vi "LinearPlntInvFF_Calculate_NextR.vi"(9 "NextR":T1, 11 "Input Linear Plant Inv FF":T2) -> (0 "Error":bool, 2 "Uff":T1, 3 "Output Linear Plant Inv FF":T2)   [LabVIEW 2019, in "Trajectory_Library.lvlib"]
doc: "Creates a new LINEAR PLANT INVERSION FEEDFORWARD data cluster with the specified values. \n\n\nInputs: \n - XXX -- XXX.\n\nOutputs:\n - XXX -- XXX."
uses:
  LINEAR_PLANT_INV_FF.ctl
  <vilib>/Analysis/Matrix/Datatypes/RealMatrix.ctl
  Trajectory_Library.lvlib
  <vilib>/Analysis/Matrix/NI_Matrix.lvlib
panel:
  # "<States,1>"
  # "<Inputs,1>"
  # "<States,Inputs>"
  # "<States,States>"
  # "<States,1>"
  # "<Inputs,1>"
  # "<States,Inputs>"
  # "<States,States>"
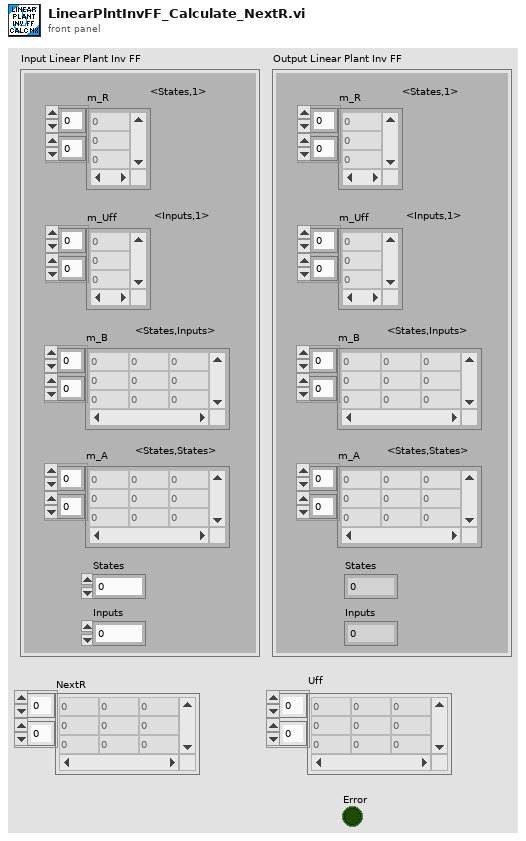
[diagram p1: front panel]
types:
  T1 = typedef "NI_Matrix.lvlib/RealMatrix.ctl" = dbl[][]
  T2 = typedef "Trajectory_Library.lvlib/LINEAR_PLANT_INV_FF.ctl" = cluster{"m_R":T1, "m_Uff":T1, "m_B":T1, "m_A":T1, "States":i32, "Inputs":i32}
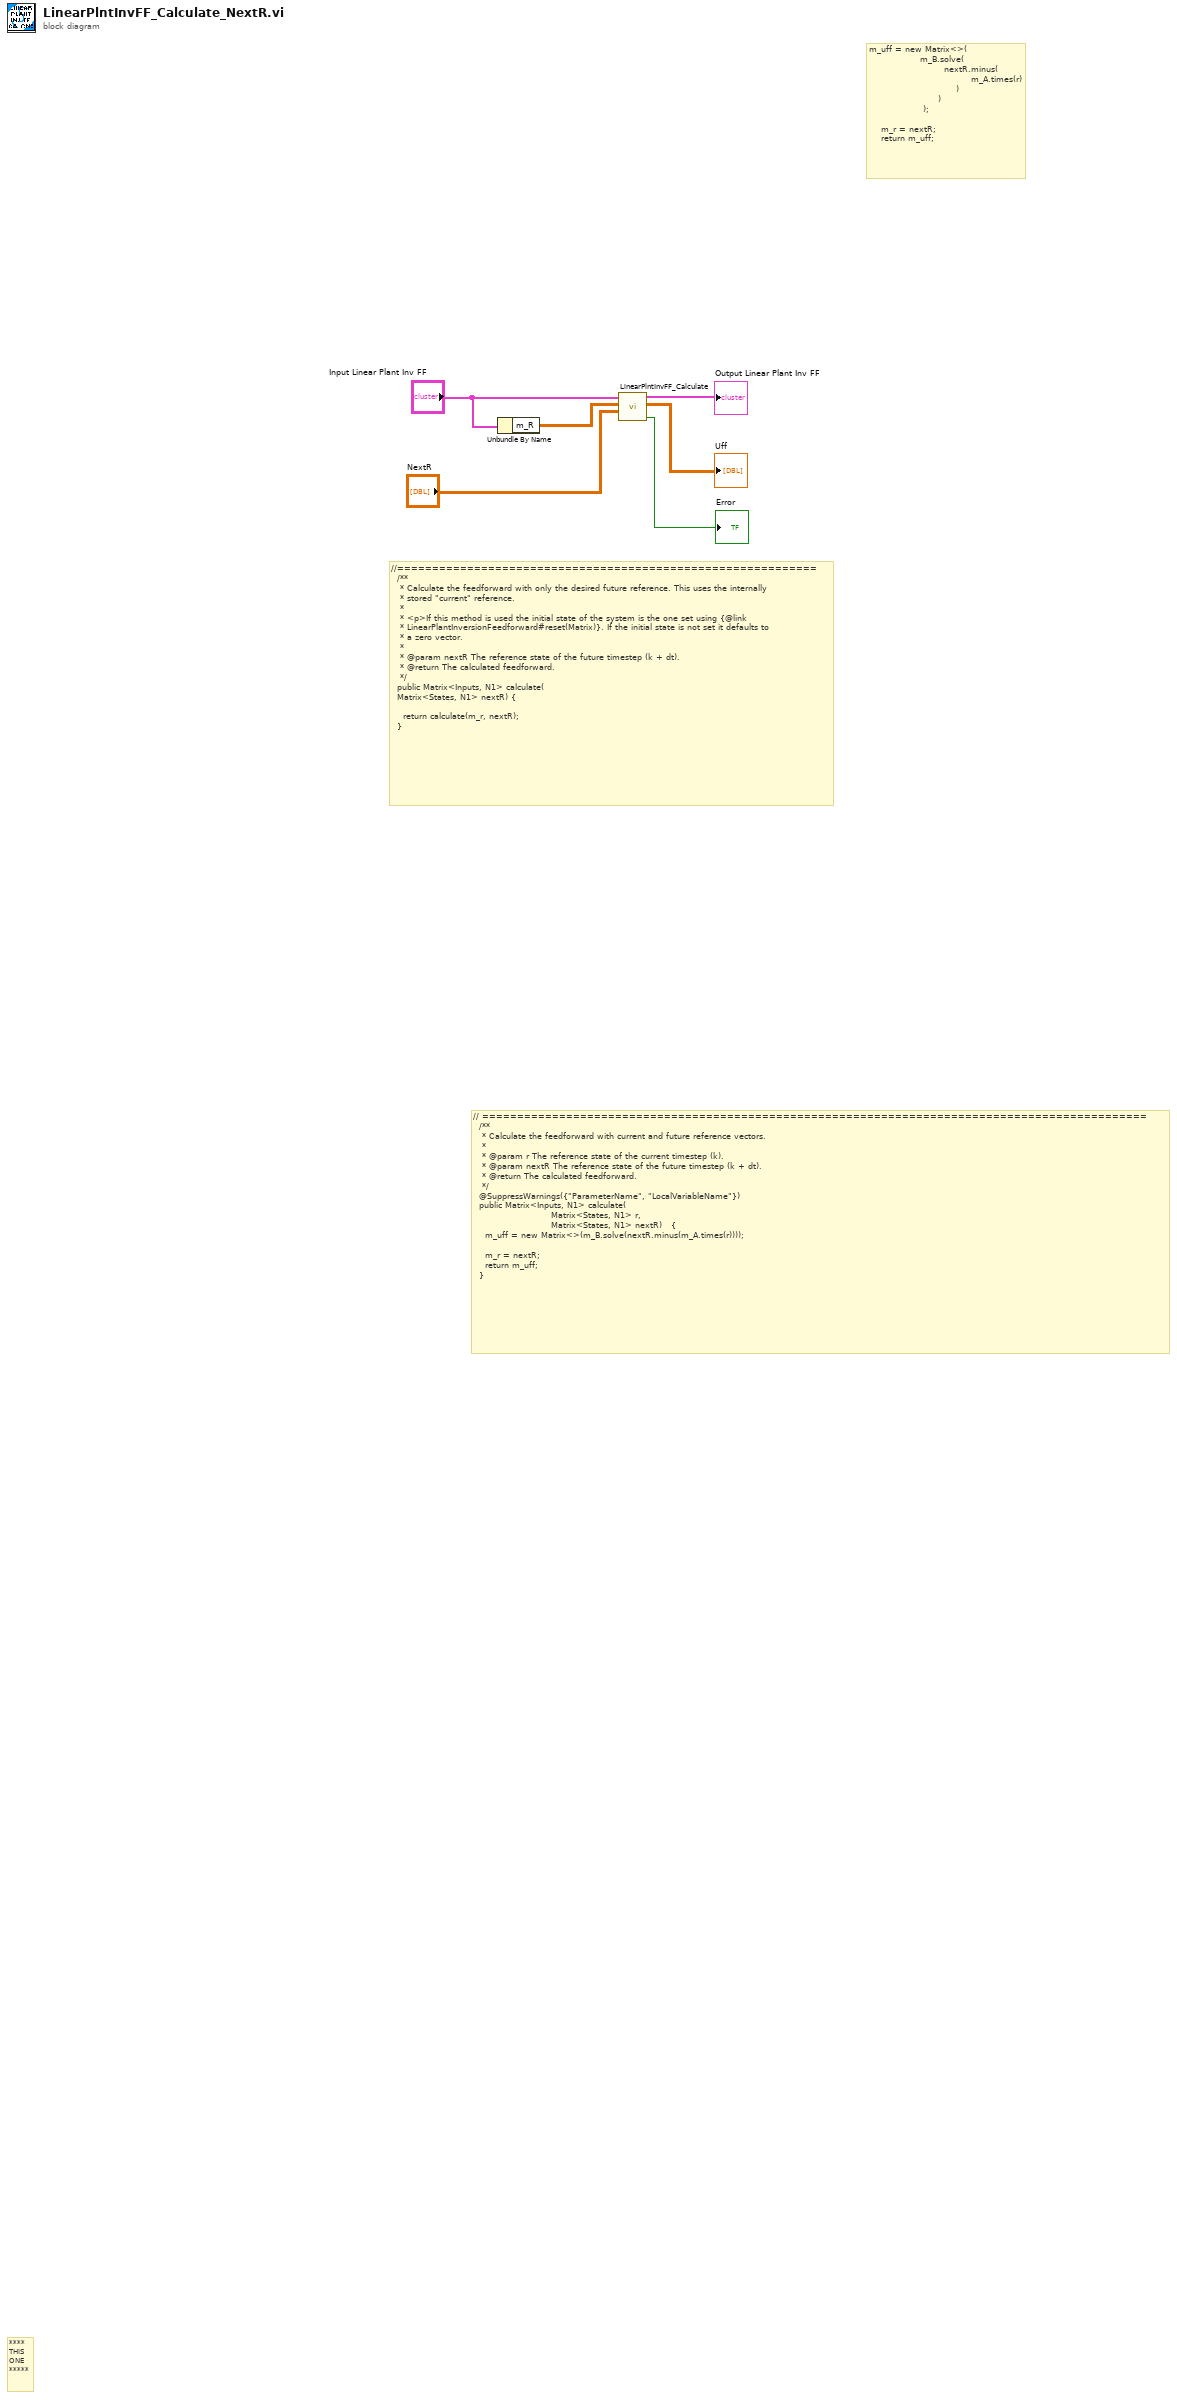
[diagram p0: block diagram]
diagram:
  # "//============================================================\n  /**\n   * Calculate the feedforward with only the desired future reference. This uses the internally\n   * stored \"current\" reference.\n   *\n   * <p>If this method is used the initial state of the system is the one set using {@link\n   * LinearPlantInversionFeedforward#reset(Matrix)}. If the initial state is not set it defaults to\n   * a zero vector.\n   *\n   * @param nextR The reference state of the future timestep (k + dt).\n   * @return The calculated feedforward.\n   */\n  public Matrix<Inputs, N1> calculate(\n\t\tMatrix<States, N1> nextR) {\n\n    return calculate(m_r, nextR);\n  }"
  # "m_uff = new Matrix<>(\n                 m_B.solve(\n                         nextR.minus(\n                                  m_A.times(r) \n                             )\n                       )\n                  );\n\n    m_r = nextR;\n    return m_uff;"
  # "// ===============================================================================================\n  /**\n   * Calculate the feedforward with current and future reference vectors.\n   *\n   * @param r The reference state of the current timestep (k).\n   * @param nextR The reference state of the future timestep (k + dt).\n   * @return The calculated feedforward.\n   */\n  @SuppressWarnings({\"ParameterName\", \"LocalVariableName\"})\n  public Matrix<Inputs, N1> calculate(\n                          Matrix<States, N1> r, \n                          Matrix<States, N1> nextR)   {\n    m_uff = new Matrix<>(m_B.solve(nextR.minus(m_A.times(r))));\n\n    m_r = nextR;\n    return m_uff;\n  }"
  # "****\nTHIS\nONE\n*****"
  n1 = Unbundle By Name("Input Linear Plant Inv FF") -> ("m_R"=w2:T1)
  n2 = call "LinearPlntInvFF_Calculate.vi"("NextR"="NextR", "R"=w2, "Input Linear Plant Inv FF"="Input Linear Plant Inv FF") -> ("Error"=→"Error":bool, "Uff"=→"Uff":T1, "Output Linear Plant Inv FF"=→"Output Linear Plant Inv FF":T2)  [unwired: 6 in]
